vi "LJM_CleanInterval.vi"(8 "error in":errorcluster, 11 "Interval Handle":i32 format="%.0g") -> (0 "error out":errorcluster)   [LabVIEW 2020]
uses:
  Library/Frameworks/LabJackM.framework
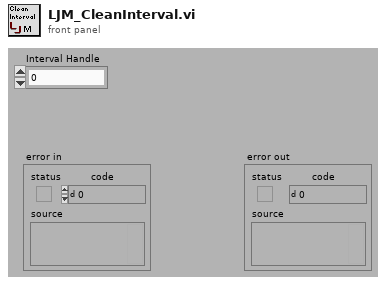
[diagram p1: front panel]
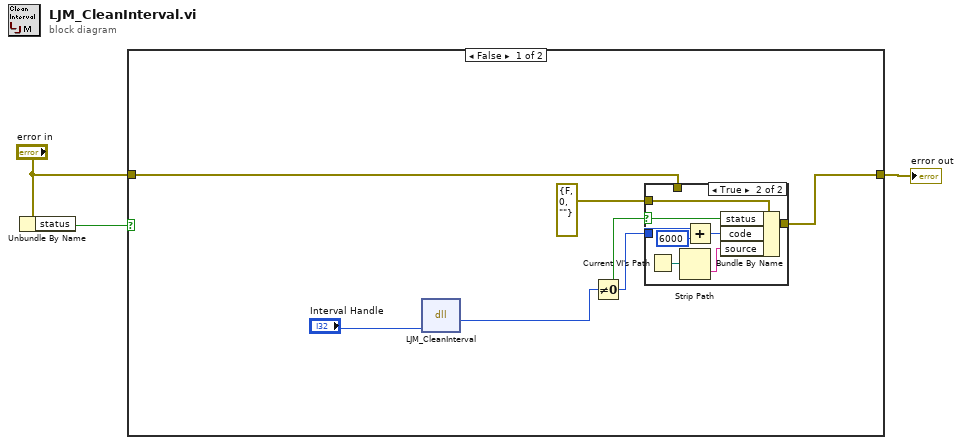
[diagram p0: block diagram]
diagram:
  n1 = Unbundle By Name("error in") -> ("status"=w1:bool)
  n2 = case shown="False" w1 {
    tunnel: "error in" -> [w7 w19]
    tunnel: [w6 w19] -> w3
    frame False {
      n3 = dll-call lib="Library/Frameworks/LabJackM.framework" fn="LJM_CleanInterval"("IntervalHandle"="Interval Handle") -> ("return type"=w5:i32)  [unwired: 4 in, 2 out]
      n4 = Not Equal To 0?(x=w5) -> (x != 0?=w9:bool)
      n5 = case shown="True" w9 {
        selector: w9 -> [_ w17]
        tunnel: [w10 w18] -> w6
        tunnel: errorcluster {"status"=FALSE, "code"=0, "source"=""} ("error IO") -> [_ w16]
        tunnel: w5 -> [_ w12]
        tunnel: w7 -> [w10 _]
        frame False {
        }
        frame True {
          n6 = Current VI's Path() -> (path=w14:path)
          n7 = Strip Path(path=w14) -> (name=w15:string)  [unwired: 1 out]
          n8 = Add(x=w12, y=6000) -> (x+y=w13:i32)
          n9 = Bundle By Name(cluster=w16, "status"=w17, "code"=w13, "source"=w15) -> (w18:errorcluster)
        }
      }
    }
    frame True {
    }
  }
  "error out" <- w3
